vi "Next Page.vi"(8 "error in (no error)":errorcluster, 11 "Project Model in":refnum<class "Project Model.lvclass">) -> (0 "error out":errorcluster, 3 "Project Model out":refnum<class "Project Model.lvclass">)   [LabVIEW 2013, in "Project Model.lvlib" / "Project Model.lvclass"]
uses:
  Project Model.lvclass
  Project Model.lvclass/Project Model.ctl
  <vilib>/ActorFrameworkMVC/View Observer/View Registry/View Registry.lvclass/View Registry.ctl
  Project Model Messages/Abstract Move In Next Msg/Abstract Move In Next Msg.lvclass
  <vilib>/ActorFrameworkMVC/View Observer/View Registry/View Registry.lvclass
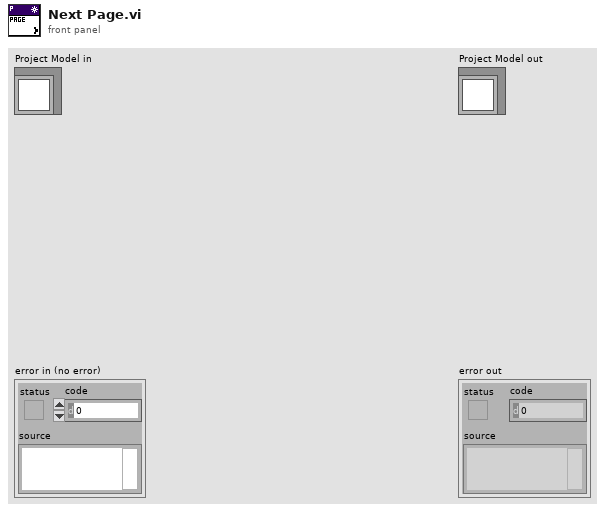
[diagram p1: front panel]
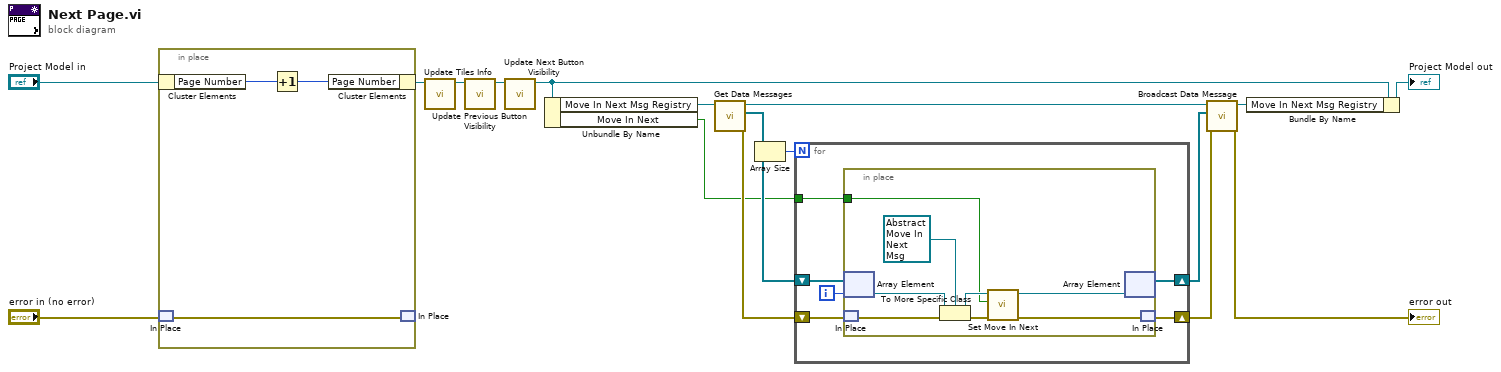
[diagram p0: block diagram]
diagram:
  n1 = in-place {
    n2 = in-place-cluster #1("Project Model in") -> ("Page Number"=w20:i32)
    n3 = in-place-match #2("error in (no error)") -> (w18:errorcluster)
    n4 = Increment(x=w20) -> (x+1=w19:i32)
    n5 = in-place-cluster #1("Page Number"=w19) -> (w4:refnum<class "Project Model.lvclass">)
    n6 = in-place-match #2(w18) -> ()  [unwired: 1 out]
  }
  n7 = call "Update Tiles Info.vi"("Project Model in"=w4) -> ("Project Model out"=w3:refnum<class "Project Model.lvclass">)  [unwired: 9 in, 1 out]
  n8 = call "Update Previous Button Visibility.vi"("Project Model in"=w3) -> ("Project Model out"=w2:refnum<class "Project Model.lvclass">)  [unwired: 9 in, 1 out]
  n9 = call "Update Next Button Visibility.vi"("Project Model in"=w2) -> ("Project Model out"=w1:refnum<class "Project Model.lvclass">)  [unwired: 9 in, 1 out]
  n10 = Unbundle By Name(w1) -> ("Move In Next Msg Registry"=w15:refnum<class "View Registry.lvclass">, "Move In Next"=w7:bool)
  n11 = call <vilib>:"Get Data Messages.vi"("View Registry in"=w15) -> ("error out"=w11:errorcluster, "Data Messages"=w12:refnum<class "Data Message.lvclass">[], "View Registry out"=w14:refnum<class "View Registry.lvclass">)  [unwired: 8 in]
  n12 = Array Size(array=w12) -> (size(s)=w13:i32)
  n13 = for {
    N: w13 -> [_]
    shift-right: [w25] -> w10
    shift-left: w12 -> [w26]
    shift-right: [w22] -> w9
    shift-left: w11 -> [w24]
    tunnel: w7 -> [w23]
    i -> [w21]
    n14 = in-place {
      in-place-border: w23 -> [w27]
      n15 = in-place-array #3(w26, w21) -> (w32:refnum<class "Data Message.lvclass">)
      n16 = in-place-match #4(w24) -> (w34:errorcluster)
      n17 = To More Specific Class(target class=refnum<class "Abstract Move In Next Msg.lvclass"> refnum ("Project Model.lvlib:Abstract Move In Next Msg.lvclass"), reference=w32, error in=w34) -> (specific class reference=w28:refnum<class "Abstract Move In Next Msg.lvclass">, error out=w31:errorcluster)
      n18 = call "Set Move In Next.vi"("error in (no error)"=w31, "Move In Next"=w27, "Abstract Move In Next Msg in"=w28) -> ("error out"=w30:errorcluster, "Abstract Move In Next Msg out"=w29:refnum<class "Abstract Move In Next Msg.lvclass">)  [unwired: 7 in]
      n19 = in-place-array #3(w29) -> (w25:refnum<class "Data Message.lvclass">[])  [unwired: 1 out]
      n20 = in-place-match #4(w30) -> (w22:errorcluster)
    }
  }
  n21 = call <vilib>:"Broadcast Data Message.vi"("error in (no error)"=w9, "Data Messages"=w10, "View Registry in"=w14) -> ("error out"=→"error out":errorcluster, "View Registry out"=w8:refnum<class "View Registry.lvclass">)  [unwired: 7 in]
  n22 = Bundle By Name(cluster=w1, "Move In Next Msg Registry"=w8) -> (→"Project Model out":refnum<class "Project Model.lvclass">)
